vi "Seek_Above50_20KHZ_Test.vi"() -> ()   [LabVIEW 2017]
panel:
  out "Error Output":errorcluster
  out "SEEK recipe Parameters range validation":string
  out "Test Result":picture
  out "Response Graph":cluster{dbl, u32}[](graph)
  # "SEEK recipe parameters range value :\n------------------------------------------ \nSeekTime=1 to 1000\nSeekAmplitudeloopC1=1 to 20000\nSeekAmplitudeLoopC2=1 to 20000\nSeekFreqLimitHigh=1 to 500 [20KHz], 1 to 750[30KHz], 1 to 1000[40KHz]\nSeekFreqLimitLow=1 to 500 [20KHz], 1 to 750[30KHz], 1 to 1000[40KHz]\nSeekPhaseloopI=50 to 500\nSeekPhaseloopCF=50 to 500\nSeekRampTime=10 to 1000\nSeekFreqOffset= 0 to 1000\nMemoryClearBeforeSeek=0 or 1"
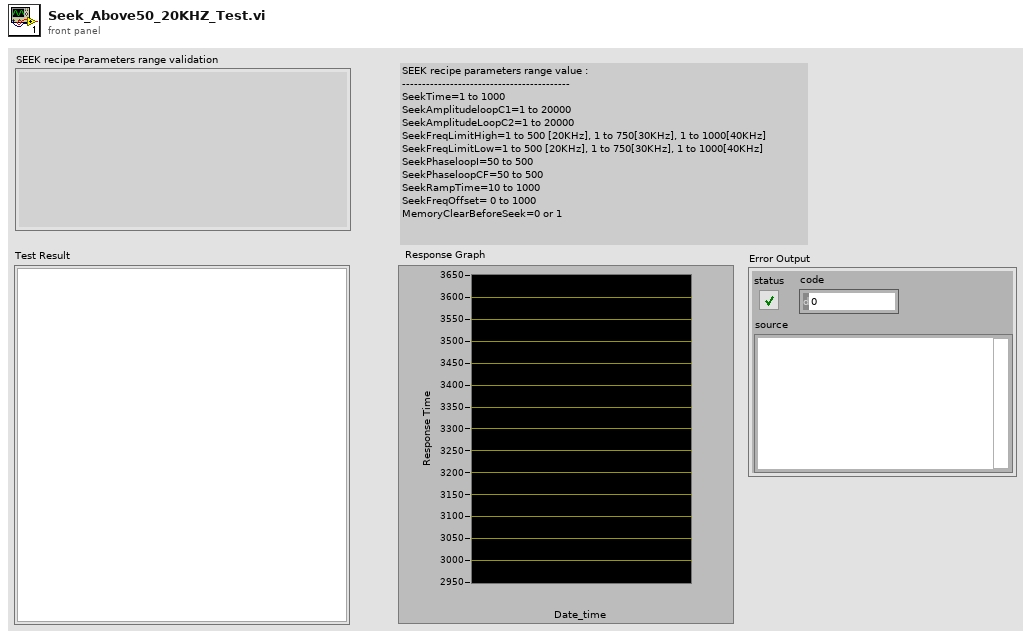
[diagram p1: front panel]
types:
  T1 = enum16{"open", "replace", "create", "open or create", "replace or create", "replace or create with confirmation"}
  T2 = cluster{"[0]":string, "[1]":string, "[2]":string, "[3]":string, "[4]":string, "[5]":string, "[6]":string, "[7]":string, "[8]":string}
  T3 = cluster{"Iterations":u64, "DelayBetweenIterations":u32, "Timeout":u32, "MessageID":i32, "MessageLength":i32, "ResponseID":i32, "SeekTime":i32, "SeekAmplitudeLoopC1":i32, "SeekAmplitudeLoopC2":i32, "SeekFreqLimitHigh":i32, "SeekFreqLimitLow":i32, "SeekPhaseloopI":i32, "SeekPhaseloopCF":i32, "SeekRampTime":i32, "SeekFreqOffset":i32, "MemoryClearBeforeSeek":i32, "Timestamp":string, "TestSuite":string, "ReportPath":path, "FWVersionPath":path}
  T4 = cluster{"Socket_IP_Address":string, "Socket_Port_Number":u16, "Global_ReportPath":path}
  T5 = typedef "imagedata.ctl" = cluster{"image type":i32, "image depth":i32, "image":u8[], "mask":u8[], "colors":u32[], "Rectangle":cluster{"left":i16, "top":i16, "right":i16, "bottom":i16}}
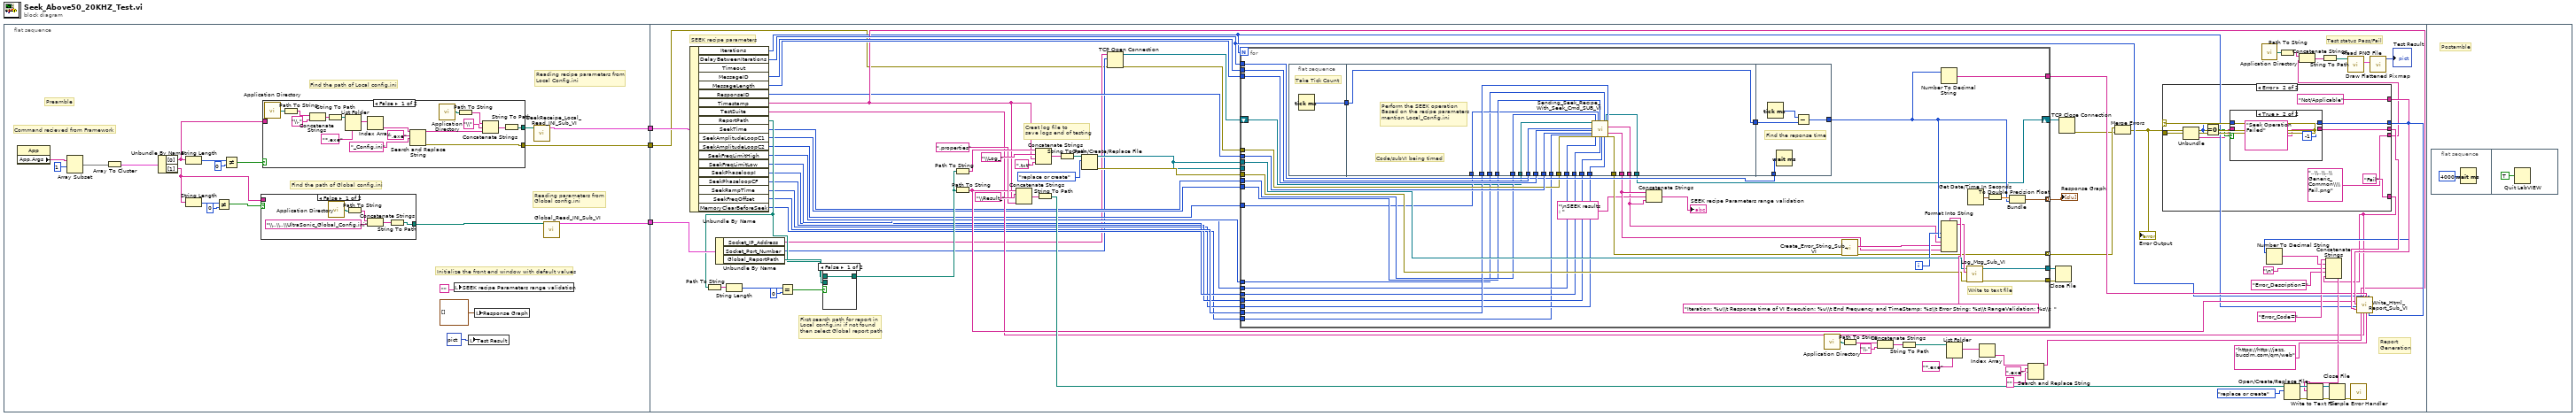
[diagram p0: block diagram]
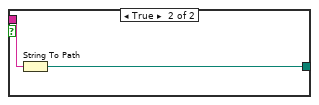
[diagram p2: hidden frame]
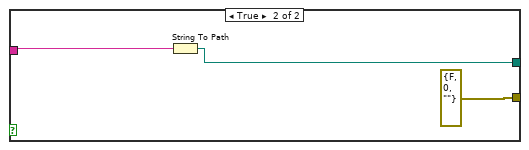
[diagram p3: hidden frame]
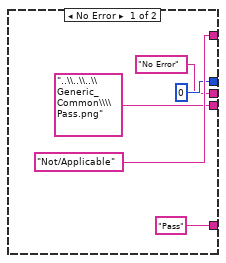
[diagram p5: hidden frame]
diagram:
  n1 = flat-sequence {
    tunnel: [w9] -> w3
    tunnel: [w8] -> w2
    tunnel: [w7] -> w1
    tunnel: w3 -> [w55]
    tunnel: w2 -> [w79]
    tunnel: w1 -> [w68]
    frame #0 {
      # "Find the path of Global config.ini"
      # "Find the path of Local config.ini"
      # "Reading parameters from \nGlobal config.ini"
      # "Reading recipe parameters from \nLocal Config.ini"
      # "Command recieved from Framework"
      # "Initialize the front end window with default values"
      # "Preamble"
      n2 = property class="App"() -> ("App.Args"=w11:string[])  [unwired: 2 in, 2 out]
      n3 = Array Subset "Array Subset"(array=w11, index=1) -> (w12:string[])  [unwired: 1 in]
      n4 = Array To Cluster(array=w12) -> (cluster=w13:T2)
      n5 = Unbundle By Name "Unbundle By Name"(w13) -> ("[0]"=w17:string, "[1]"=w20:string)
      n6 = String Length(string=w20) -> (length=w21:i32)
      n7 = String Length(string=w17) -> (length=w14:i32)
      n8 = Not Equal?(x=w21, y=0) -> (x != y?=w19:bool)
      n9 = Not Equal?(x=w14, y=0) -> (x != y?=w16:bool)
      n10 = case shown="False" w19 {
        tunnel: [w25 w30] -> w23
        tunnel: w20 -> [_ w29]
        frame False {
          n11 = call <vilib>:"Application Directory.vi"() -> ("Application Directory"=w24:path)
          n12 = Path To String(path=w24) -> (string=w28:string)
          n13 = Concatenate Strings(w28, "\\..\\..\\UltraSonic_Global_Config.ini" ("string")) -> (w26:string)
          n14 = String To Path(string=w26) -> (path=w25:path)
        }
        frame True {
          n15 = String To Path(string=w29) -> (path=w30:path)
        }
      }
      n16 = case shown="False" w16 {
        tunnel: w17 -> [_ w50]
        tunnel: [w32 w49] -> w22
        tunnel: [w31 errorcluster {"status"=FALSE, "code"=0, "source"=""} ("error out")] -> w9
        frame False {
          n17 = call <vilib>:"Application Directory.vi"() -> ("Application Directory"=w38:path)
          n18 = Path To String(path=w38) -> (string=w37:string)
          n19 = Concatenate Strings(w37, "\\." ("string")) -> (w35:string)
          n20 = String To Path(string=w35) -> (path=w40:path)
          n21 = List Folder(path=w40, pattern="*.exe") -> (filenames=w34:string[])  [unwired: 2 in, 3 out]
          n22 = Index Array(array=w34) -> (element=w33:string)  [unwired: 1 in]
          n23 = Search and Replace String(input string=w33, search string=".exe", replace string="_Config.ini" ("replace string (\"\")")) -> (result string=w44:string, error out=w31:errorcluster)  [unwired: 5 in, 2 out]
          n24 = call <vilib>:"Application Directory.vi"() -> ("Application Directory"=w47:path)
          n25 = Path To String(path=w47) -> (string=w42:string)
          n26 = Concatenate Strings(w42, "\\" ("string"), w44) -> (w41:string)
          n27 = String To Path(string=w41) -> (path=w32:path)
        }
        frame True {
          n28 = String To Path(string=w50) -> (path=w49:path)
        }
      }
      n29 = local write "SEEK recipe Parameters range validation"("") -> ()
      n30 = local write "Test Result"(picture data[5B] ("Test Result")) -> ()
      n31 = local write "Response Graph"(cluster{dbl, u32}[] [] ("Response Graph")) -> ()
      n32 = call "SeekReceipe_Local_Read_INI_Sub_VI.vi"("Config File Path"=w22) -> ("Content from ini file"=w7:T3)  [unwired: 9 in]
      n33 = call "Global_Read_INI_Sub_VI.vi"("Config File Path"=w23) -> ("output cluster"=w8:T4)  [unwired: 14 in]
    }
    frame #1 {
      # "Creat log file to \nsave logs end of testing"
      # "First search path for report in\nLocal config.ini if not found\nthen select Global report path"
      # "Test status Pass/Fail"
      # "Report \nGeneration"
      # "SEEK recipe parameters"
      n34 = Unbundle By Name(w68) -> ("Iterations"=w71:u64, "DelayBetweenIterations"=w75:u32, "MessageID"=w77:i32, "MessageLength"=w76:i32, "ResponseID"=w69:i32, "Timestamp"=w73:string, "TestSuite"=w72:string, "ReportPath"=w70:path, "SeekTime"=w66:i32, "SeekAmplitudeLoopC1"=w65:i32, "SeekAmplitudeLoopC2"=w64:i32, "SeekFreqLimitHigh"=w63:i32, "SeekFreqLimitLow"=w62:i32, "SeekPhaseloopI"=w61:i32, "SeekPhaseloopCF"=w60:i32, "SeekRampTime"=w59:i32, "SeekFreqOffset"=w67:i32, "MemoryClearBeforeSeek"=w58:i32)  [unwired: 1 out]
      n35 = Path To String(path=w70) -> (string=w126:string)
      n36 = Unbundle By Name(w79) -> ("Socket_IP_Address"=w57:string, "Socket_Port_Number"=w56:u16, "Global_ReportPath"=w78:path)
      n37 = String Length(string=w126) -> (length=w125:i32)
      n38 = Equal?(x=w125, y=0) -> (x = y?=w123:bool)
      n39 = case shown="False" w123 {
        tunnel: w78 -> [_ w138]
        tunnel: [w137 w138] -> w122
        tunnel: w70 -> [w137 _]
        frame False {
        }
        frame True {
        }
      }
      n40 = Path To String(path=w122) -> (string=w128:string)
      n41 = Path To String(path=w122) -> (string=w99:string)
      n42 = Concatenate Strings(w99, "\\Result_" ("string"), w73, ".properties" ("string")) -> (w120:string)
      n43 = Concatenate Strings(w128, "\\Log_" ("string"), w73, ".txt" ("string")) -> (w131:string)
      n44 = String To Path(string=w120) -> (path=w112:path)
      n45 = String To Path(string=w131) -> (path=w130:path)
      n46 = Open/Create/Replace File(file path (use dialog)=w130, operation (0:open)=T1."replace or create") -> (refnum out=w100:refnum<file>, error out=w103:errorcluster)  [unwired: 1 in, 4 out]
      n47 = TCP Open Connection(address=w57, remote port or service name=w56, error in (no error)=w55) -> (connection ID=w52:refnum<k5>, error out=w54:errorcluster)  [unwired: 2 in]
      n48 = for {
        N: w71 -> [_]
        tunnel: [w174] -> w134
        tunnel: w100 -> [w168]
        tunnel: [w167] -> w102
        tunnel: [w165] -> w101
        tunnel: [w170] -> w132 mode=indexing
        tunnel: w103 -> [w166]
        tunnel: w100 -> [_]
        tunnel: [w162] -> w98 mode=indexing
        tunnel: w77 -> [w161]
        tunnel: w76 -> [w160]
        tunnel: w69 -> [w159]
        tunnel: w75 -> [w158]
        tunnel: w54 -> [w156]
        tunnel: w67 -> [w155]
        tunnel: w66 -> [w154]
        tunnel: w65 -> [w153]
        tunnel: w64 -> [w152]
        tunnel: w63 -> [w151]
        tunnel: w62 -> [w150]
        tunnel: w61 -> [w149]
        tunnel: w60 -> [w148]
        tunnel: w59 -> [w147]
        tunnel: w58 -> [w145]
        shift-right: [w144] -> w53
        shift-left: w52 -> [w143]
        i -> [w163]
        # "Write to text file"
        n49 = flat-sequence {
          tunnel: [w177] -> w176
          tunnel: [w197] -> w175
          tunnel: w176 -> [w197]
          tunnel: w161 -> [w196]
          tunnel: w160 -> [w195]
          tunnel: w159 -> [w194]
          tunnel: w156 -> [w193]
          tunnel: w155 -> [w192]
          tunnel: w154 -> [w191]
          tunnel: w153 -> [w190]
          tunnel: w152 -> [w189]
          tunnel: w151 -> [w188]
          tunnel: w150 -> [w187]
          tunnel: w149 -> [w186]
          tunnel: w148 -> [w185]
          tunnel: w147 -> [w184]
          tunnel: [w178] -> w140
          tunnel: [w183] -> w146
          tunnel: w145 -> [w182]
          tunnel: w143 -> [w181]
          tunnel: [w180] -> w144
          tunnel: [w179] -> w142
          tunnel: w175 -> [w201]
          tunnel: [w199] -> w164
          tunnel: w158 -> [w198]
          frame #0 {
            # "Take Tick Count"
            n50 = Tick Count (ms)() -> (millisecond timer value=w177:u32)
          }
          frame #1 {
            # "Perform the SEEK operation\nBased on the recipe parameters\nmention Local_Config.ini"
            # "Code/subVI being timed"
            n51 = call "Sending_Seek_Recipe_With_Seek_Cmd_SUB_VI.vi"("connection ID - In"=w181, "Receipe Msg ID"=w196, "Receipe Message length"=w195, "Response ID"=w194, "MemoryClearBeforeSeek"=w182, "error in (no error)"=w193, "SeekTime"=w191, "SeekFreqLimitLow"=w187, "SeekAmplitudeLoopC2"=w189, "SeekAmplitudeLoopC1"=w190, "SeekPhaseloopI"=w186, "SeekPhaseloopCF"=w185, "SeekFreqLimitHigh"=w188, "SeekRampTime"=w184, "SeekFreqOffset"=w192) -> ("connection ID out"=w180:refnum<k5>, "End Frequency and Time Stamp"=w178:string, "SEEK recipe Parameter range validation"=w179:string, "error out"=w183:errorcluster)  [unwired: 9 in]
          }
          frame #2 {
            # "Find the reponse time"
            n52 = Tick Count (ms)() -> (millisecond timer value=w200:u32)
            n53 = Wait (ms)(milliseconds to wait=w198) -> ()  [unwired: 1 out]
            n54 = Subtract(x=w200, y=w201) -> (x-y=w199:u32)
          }
        }
        n55 = Concatenate Strings(w142, "\nSEEK results : " ("string"), w140) -> (→"SEEK recipe Parameters range validation":string)
        n56 = call "Create_Error_String_Sub_VI.vi"("error in"=w146) -> ("error out"=w162:errorcluster, "Error String"=w157:string)  [unwired: 9 in]
        n57 = Number To Decimal String(number=w164) -> (decimal integer string=w174:string)  [unwired: 1 in]
        n58 = Format Into String(format string="Iteration: %u\\t Response time of VI Execution: %u\\t End Frequency and TimeStamp: %s\\t Error String: %s\\t RangeValidation: %s\\t  ", w163, w164, w140, w157, w142) -> (resulting string=w169:string)  [unwired: 2 in, 1 out]
        n59 = call "Log_Msg_Sub_VI.vi"("error in (no error)"=w166, "String"=w169, "Byte Stream File in"=w168) -> ("error out"=w165:errorcluster, "Byte Stream File out"=w167:refnum<file>)  [unwired: 7 in]
        n60 = Get Date/Time In Seconds() -> (seconds since 1Jan1904=w171:timestamp)
        n61 = To Double Precision Float(number=w171) -> (double precision float=w172:dbl)
        n62 = Bundle "Bundle"(w172, w164) -> (w170:cluster{dbl, u32})  [unwired: 1 in]
      }
      "Response Graph" <- w132
      n63 = call <vilib>:"Application Directory.vi"() -> ("Application Directory"=w95:path)
      n64 = Path To String(path=w95) -> (string=w94:string)
      n65 = Concatenate Strings(w94, "\\." ("string")) -> (w92:string)
      n66 = String To Path(string=w92) -> (path=w97:path)
      n67 = List Folder(path=w97, pattern="*.exe") -> (filenames=w91:string[])  [unwired: 2 in, 3 out]
      n68 = Index Array(array=w91) -> (element=w87:string)  [unwired: 1 in]
      n69 = Search and Replace String(input string=w87, search string=".exe", replace string="" ("replace string (\"\")")) -> (result string=w90:string)  [unwired: 5 in, 3 out]
      n70 = Close File(refnum=w102, error in=w101) -> ()  [unwired: 2 out]
      n71 = TCP Close Connection(connection ID=w53) -> (error out=w51:errorcluster)  [unwired: 2 in, 1 out]
      n72 = Merge Errors "Merge Errors"(w98, w51) -> (w74:errorcluster)
      "Error Output" <- w74
      n73 = case shown="Error" w74 {
        tunnel: ["Pass" "Fail"] -> w104
        tunnel: w74 -> [_ w213]
        tunnel: [0 ("code") w209] -> w108
        tunnel: ["No Error" ("source") w210] -> w136
        tunnel: ["Not/Applicable" "Not/Applicable"] -> w135
        tunnel: ["..\\..\\..\\Generic_Common\\\\Pass.png" ("string") "..\\..\\..\\Generic_Common\\\\Fail.png" ("string")] -> w80
        frame No Error {
        }
        frame Error {
          n74 = Unbundle(w213) -> ("code"=w211:i32, "source"=w207:string)  [unwired: 1 out]
          n75 = Equal To 0?(x=w211) -> (x = 0?=w208:bool)
          n76 = case shown="True" w208 {
            tunnel: [w217 -1 ("code")] -> w209
            tunnel: [w216 "Seek Operation Failed" ("source")] -> w210
            tunnel: w211 -> [w217 _]
            tunnel: w207 -> [w216 _]
            frame False {
            }
            frame True {
            }
          }
        }
      }
      n77 = call <vilib>:"Application Directory.vi"() -> ("Application Directory"=w81:path)
      n78 = Number To Decimal String(number=w108) -> (decimal integer string=w107:string)  [unwired: 1 in]
      n79 = Path To String(path=w81) -> (string=w82:string)
      n80 = Open/Create/Replace File(file path (use dialog)=w112, operation (0:open)=T1."replace or create") -> (refnum out=w111:refnum<file>, error out=w116:errorcluster)  [unwired: 4 in, 1 out]
      n81 = Concatenate Strings(w82, w80) -> (w83:string)
      n82 = String To Path(string=w83) -> (path=w86:path)
      n83 = Concatenate Strings("Error_Code=" ("string"), w107, "\n", "Error_Description=" ("string"), w104) -> (w110:string)
      n84 = Write to Text File(file (use dialog)=w111, text=w110, error in=w116) -> (refnum out=w115:refnum<file>, error out=w114:errorcluster)  [unwired: 1 in, 1 out]
      n85 = Close File(refnum=w115, error in=w114) -> (error out=w113:errorcluster)  [unwired: 1 out]
      n86 = call <vilib>:"Read PNG File.vi"("path to PNG file"=w86) -> ("image data"=w84:T5)  [unwired: 8 in, 2 out]
      n87 = call <vilib>:"Simple Error Handler.vi"("error in (no error)"=w113) -> ()  [unwired: 4 in, 5 out]
      n88 = call "Write_Html_Report_Sub_VI.vi"("ReprtPath"=w99, "Remarks"=w135, "Iterations"=w71, "Error Description"=w136, "Timestamp"=w73, "TestCase"=w90, "Verdict"=w104, "TestSuite"=w72, "Time taken to execute  test in msec"=w134, "JazzDashboardLink"="https://http://jazz.bucclm.com/qm/web" ("TestSuite"), "Delay Between Iterations"=w75, "Error Code"=w108) -> ()  [unwired: 8 in]
      n89 = call <vilib>:"Draw Flattened Pixmap.vi"("image data"=w84) -> ("new picture"=→"Test Result":picture)  [unwired: 8 in]
    }
    frame #2 {
      # "Postamble"
      n90 = flat-sequence {
        frame #0 {
          n91 = Wait (ms)(milliseconds to wait=u32 4000) -> ()  [unwired: 1 out]
        }
        frame #1 {
          n92 = Quit LabVIEW(quit? (T)=TRUE) -> ()
        }
      }
    }
  }
